vi "Record IK reason.vi"(4 "reference 4":refnum<vi>, 6 "IK Reason array reference 3":refnum<vi>, 7 "Sonde IK Recording Failure Path":path, 9 "IK reference 5":refnum<vi>, 10 "reference in":refnum<vi>, 11 "Cluster 2":refnum<vi>) -> (3 "IK Reason array":string[][](array[string]))   [LabVIEW 2016]
uses:
  activeXtest/activeXtest 2015 Folder/sample data row cluster.ctl
  activeXtest/activeXtest 2015 Folder/sonde cluster.ctl
  <vilib>/Utility/file.llb/Write Delimited Spreadsheet (string).vi
panel:
  in  "Cluster":T1={"Head\nPressure"=0.0, "Depth"=0.0, "comment "="", "Sonde Data Cluster"={"Cumulative\nVolume (ml)"=100.0, "Specific\nCond (mS)"=2.0, "Dissolved\nOxygen mg/L"=3.0, "pH"=4.0, "ORP"=5.0, "Temp deg C"=26.0, "Salinity"=7.0, "Dissolved\nOxygen %"=0.0}, "Aux1"=0.0, "Aux2"=0.0, "Aux3\\EC"=0.0} {"Sonde Data Cluster"."Dissolved\nOxygen %" format="%_4g"; "Sonde Data Cluster"."Salinity" format="%_3g"; "Sonde Data Cluster"."Temp deg C" format="%_2g"; "Sonde Data Cluster"."ORP" format="%_4g"; "Sonde Data Cluster"."pH" format="%_4g"; "Sonde Data Cluster"."Dissolved\nOxygen mg/L" format="%_4g"; "Sonde Data Cluster"."Specific\nCond (mS)" format="%_4g"; "Sonde Data Cluster"."Cumulative\nVolume (ml)" format="%#_4g"}
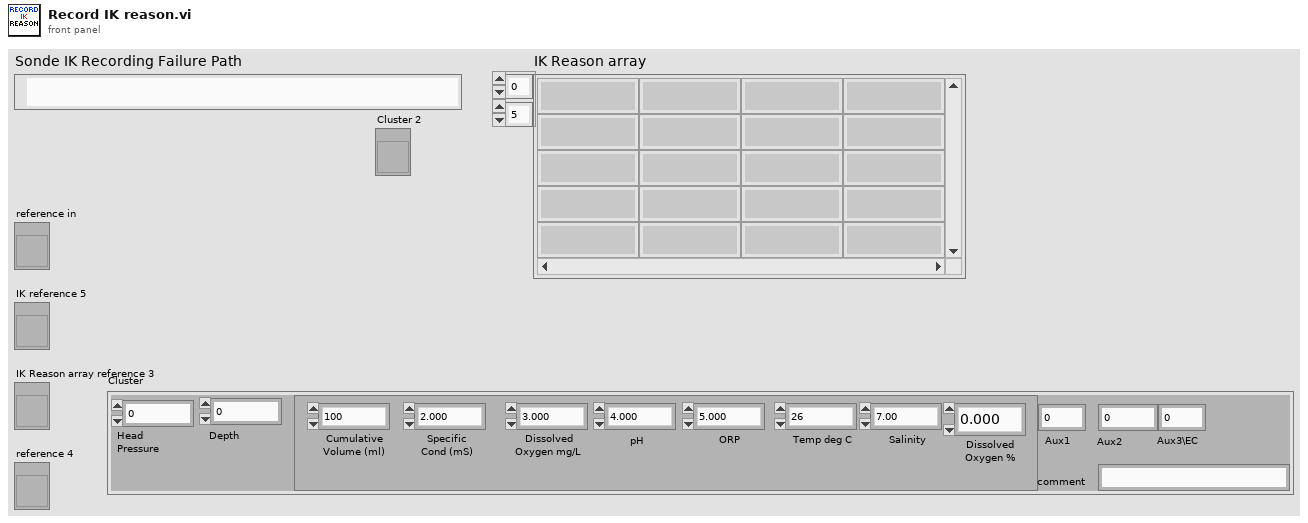
[diagram p1: front panel]
types:
  T1 = typedef "sample data row cluster.ctl" = cluster{"Head\nPressure":dbl, "Depth":dbl, "comment ":string, "Sonde Data Cluster":T2, "Aux1":dbl, "Aux2":dbl, "Aux3\\EC":dbl}
  T2 = typedef "sonde cluster.ctl" = cluster{"Cumulative\nVolume (ml)":dbl, "Specific\nCond (mS)":dbl, "Dissolved\nOxygen mg/L":dbl, "pH":dbl, "ORP":dbl, "Temp deg C":dbl, "Salinity":dbl, "Dissolved\nOxygen %":dbl}
  T3 = typedef "SS Control 7.ctl" = cluster{"Flow":dbl, "Zeroed \nPressure":dbl, "Ik":dbl, "Current Depth":sgl, "Feet of Stainless":i32, "Start Depth":sgl, "Abs Start Depth":sgl}
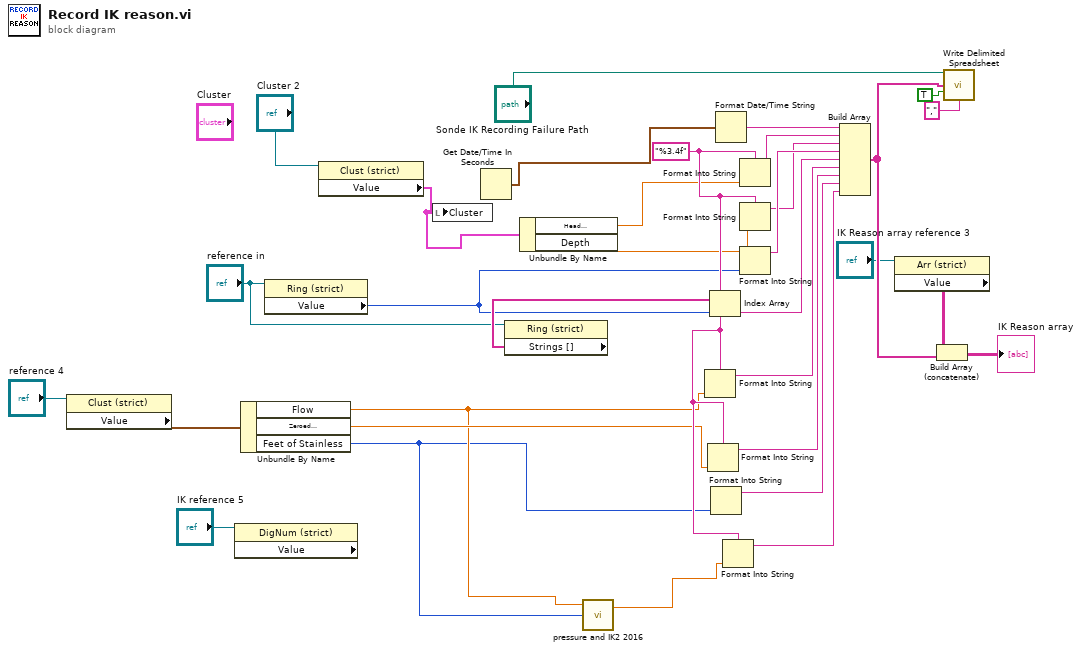
[diagram p0: block diagram]
diagram:
  w32 = "%3.4f" ("format string")
  n1 = property class="Clust (strict)"(reference="reference 4") -> ("Value"=w26:T3)  [unwired: 1 in, 2 out]
  n2 = property class="DigNum (strict)" props=["Value"](reference="IK reference 5") -> ()  [unwired: 1 in, 3 out]
  n3 = Unbundle By Name(w26) -> ("Flow"=w3:dbl, "Zeroed \nPressure"=w28:dbl, "Feet of Stainless"=w2:i32)
  n4 = property class="Ring (strict)"(reference="reference in") -> ("Value"=w21:u16)  [unwired: 1 in, 2 out]
  n5 = property class="Clust (strict)"(reference="Cluster 2") -> ("Value"=w5:T1)  [unwired: 1 in, 2 out]
  n6 = local write "Cluster"(w5) -> ()
  n7 = Get Date/Time In Seconds() -> (seconds since 1Jan1904=w10:timestamp)
  n8 = property on="Property Node" class="Ring (strict)"(reference="reference in") -> ("Strings []"=w22:string[])  [unwired: 1 in, 2 out]
  n9 = Unbundle By Name(w5) -> ("Head\nPressure"=w11:dbl, "Depth"=w12:dbl)
  n10 = call "pressure and IK2 2016.vi"("Ft. of SS"=w2, "flow"=w3) -> ("IK"=w1:dbl)  [unwired: 1 in, 1 out]
  n11 = Format Into String(format string=w32, w3) -> (resulting string=w27:string)  [unwired: 2 in, 1 out]
  n12 = Format Into String(format string=w32, w28) -> (resulting string=w29:string)  [unwired: 2 in, 1 out]
  n13 = Index Array(array=w22, index=w21) -> (element=w18:string)
  n14 = Format Into String(w2) -> (resulting string=w30:string)  [unwired: 3 in, 1 out]
  n15 = Format Date/Time String(seconds (now)=w10) -> (date/time string=w14:string)  [unwired: 2 in]
  n16 = Format Into String(format string=w32, w1) -> (resulting string=w31:string)  [unwired: 2 in, 1 out]
  n17 = Format Into String(format string=w32, w11) -> (resulting string=w15:string)  [unwired: 2 in, 1 out]
  n18 = Format Into String(format string=w32, w12) -> (resulting string=w16:string)  [unwired: 2 in, 1 out]
  n19 = Format Into String(w21) -> (resulting string=w17:string)  [unwired: 3 in, 1 out]
  n20 = Build Array(w14, w15, w16, w17, w18, w27, w29, w30, w31) -> (w19:string[])
  n21 = property class="Arr (strict)"(reference="IK Reason array reference 3") -> ("Value"=w25:string[][])  [unwired: 1 in, 2 out]
  n22 = Build Array (concatenate)(w25, w19) -> (→"IK Reason array":string[][])
  n23 = call-poly <vilib>:"Write Delimited Spreadsheet.vi"("file path (dialog if empty)"="Sonde IK Recording Failure Path", "1D data"=w19, "append to file? (new file:F)"=TRUE, "delimiter (\\t)"="," ("delimiter (\\t)")) -> ()  [unwired: 10 in, 2 out]
